vi "InitPort.vi"(9 "CONFIGURATION CLUSTER":T1) -> (0 "LV ERROR OUT":errorcluster, 2 "DUP VISA RESOURCE":refnum<visa-resource-name>="COM1", 3 "UNMODIFIED CONFIGURATION CLUSTER":T1)   [LabVIEW 2012]
doc: "This VI opens a VISA session for the serial port or serial-converted USB port indicated by the \"VISA resource\" input. Use this VISA session for all VIs in the application. Close the session by using GoLocal.vi when your application VI terminates."
uses:
  <vilib>/Instr/_visa.llb/VISA Configure Serial Port (Serial Instr).vi
panel:
  # "InitPort.vi"
  # "This VI opens a VISA session for the serial port or serial-converted USB port indicated by the \"VISA resource\" input. Use this VISA session for all VIs in the application. Close the session by using GoLocal.vi when your application VI terminates."
  # "RV-Elektroniikka Oy\nPicowatt"
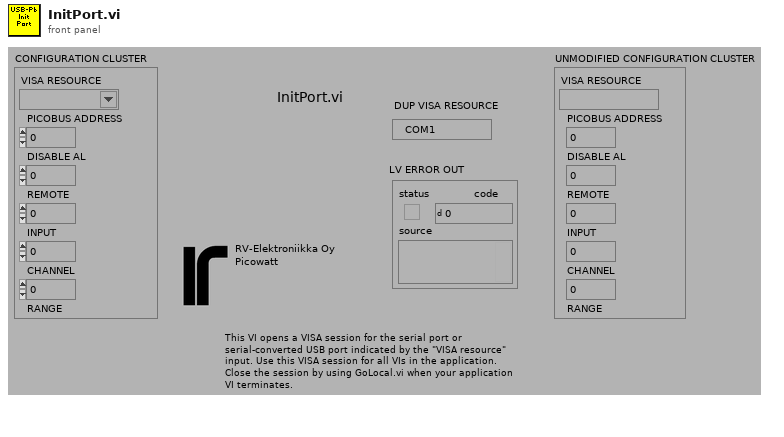
[diagram p1: front panel]
types:
  T1 = cluster{"VISA RESOURCE":refnum<visa-resource-name>, "PICOBUS ADDRESS":u8, "DISABLE AL":u8, "REMOTE":u8, "INPUT":u8, "CHANNEL":u8, "RANGE":u8, "EXCITATION":u8, "DISPLAY":u8, "DIGITAL REFERENCE":u16, "SET POINT":dbl, "PROP GAIN":u8, "INTG":u8, "DERIV":u8, "POWER BIAS":u8, "POWER RANGE":u8, "INFO STRING":string, "HEATER RESISTANCE":dbl, "INTERVAL":u8, " SENSOR dR/dT":u8}
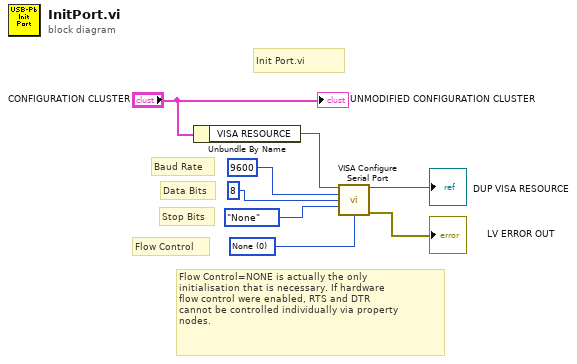
[diagram p0: block diagram]
diagram:
  w5 = u16 0 items=["None", "XON/XOFF", "RTS/CTS", "XON/XOFF & RTS/CTS", "DTR/DSR", "XON/XOFF & DTR/DSR"] ("flow control (0:none)")
  # "Flow Control=NONE is actually the only\ninitialisation that is necessary. If hardware\nflow control were enabled, RTS and DTR\ncannot be controlled individually via property\nnodes."
  # "Init Port.vi"
  # "Flow Control"
  # "Stop Bits"
  # "Data Bits"
  # "Baud Rate"
  n1 = Unbundle By Name("CONFIGURATION CLUSTER") -> ("VISA RESOURCE"=w2:refnum<visa-resource-name>)
  n2 = call-poly "VISA Configure Serial Port"("VISA resource name"=w2, "baud rate (9600)"=u32 9600, "data bits (8)"=u16 8, "parity (0:none)"=enum16{"None", "Odd", "Even", "Mark", "Space"}."None", "flow control (0:none)"=w5) -> ("VISA resource name out"=→"DUP VISA RESOURCE":refnum<visa-resource-name>, "error out"=→"LV ERROR OUT":errorcluster)  [unwired: 9 in]
  "UNMODIFIED CONFIGURATION CLUSTER" <- "CONFIGURATION CLUSTER"
